vi "Get Control Information.vi"(8 "error in (no error)":errorcluster, 11 "Control Info in":refnum<class "Control Info.lvclass">) -> (0 "error out":errorcluster, 2 "Control Information":string[][](array[string]), 3 "Control Info out":refnum<class "Control Info.lvclass">)   [LabVIEW 2017, in "Localization.lvlib" / "Control Info.lvclass"]
doc: "VI for override that is supposed to do go throgh the process for each control type and pull out the information that is necessary for each control.\n\nChoose Movement Consulting, LLC"
uses:
  Control Info.lvclass
  Control Info.lvclass/Control Info.ctl
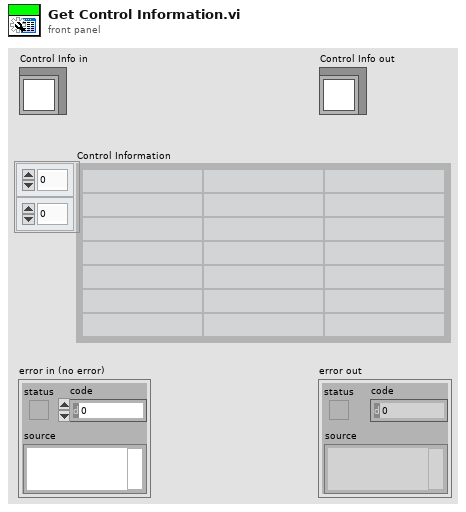
[diagram p1: front panel]
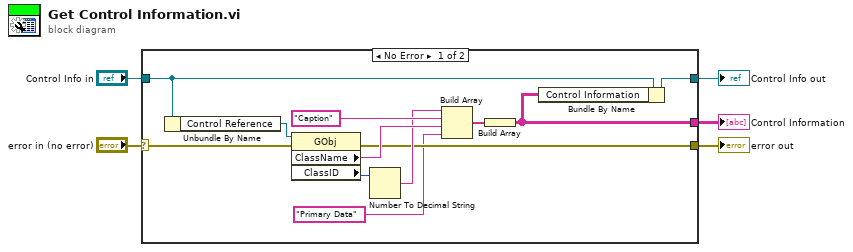
[diagram p0: block diagram]
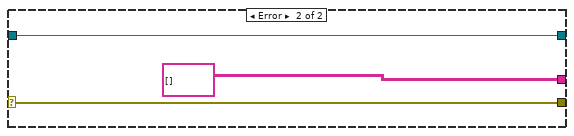
[diagram p2: hidden frame]
diagram:
  n1 = case shown="No Error" "error in (no error)" {
    selector: "error in (no error)" -> [w10 w20]
    tunnel: [w9 w20] -> w4
    tunnel: [w17 w19] -> w2
    tunnel: "Control Info in" -> [w8 w19]
    tunnel: [w11 string[][] [] ("Control Information")] -> w1
    frame No Error {
      n2 = Unbundle By Name(w8) -> ("Control Reference"=w7:refnum<vi>)
      n3 = property class="GObj"(reference=w7, error in=w10) -> (error out=w9:errorcluster, "ClassName"=w15:string, "ClassID"=w13:u32)  [unwired: 1 out]
      n4 = Number To Decimal String(number=w13) -> (decimal integer string=w12:string)  [unwired: 1 in]
      n5 = Build Array(w12, "Caption", w15, "Primary Data") -> (w14:string[])
      n6 = Build Array(w14) -> (w11:string[][])
      n7 = Bundle By Name(cluster=w8, "Control Information"=w11) -> (w17:refnum<class "Control Info.lvclass">)
    }
    frame Error {
    }
  }
  "error out" <- w4
  "Control Info out" <- w2
  "Control Information" <- w1
